vi "Time Left Calc.vi"(7 "Enum":T1, 8 "error in (no error)":errorcluster, 11 "Time":u32) -> (0 "error out":errorcluster, 2 "Time Left":u32, 3 "Total time":u32)   [LabVIEW 2018]
uses:
  Time elapsed.ctl
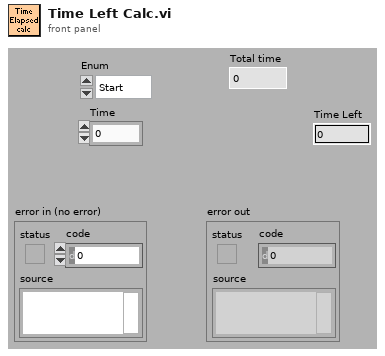
[diagram p1: front panel]
types:
  T1 = typedef "Time elapsed.ctl" = enum16{"Start", "Update", "Read"}
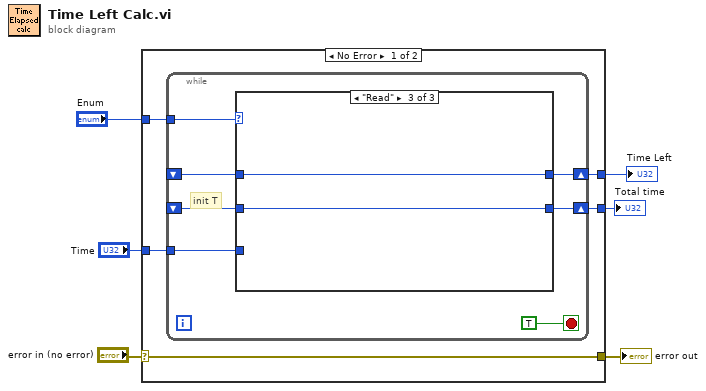
[diagram p0: block diagram]
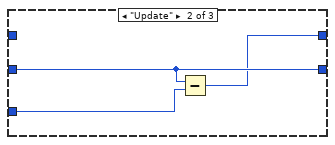
[diagram p3: hidden frame]
diagram:
  n1 = case shown="No Error" "error in (no error)" {
    selector: "error in (no error)" -> [w11 w25]
    tunnel: [w11 w25] -> w5
    tunnel: "Time" -> [w10 _]
    tunnel: [w9 _] -> w3
    tunnel: "Enum" -> [w8 _]
    tunnel: [w7 _] -> w1
    frame No Error {
      n2 = while {
        shift-right: [w12] -> w7
        shift-left: _ -> [w17]
        tunnel: w10 -> [w16]
        tunnel: w8 -> [w14]
        shift-right: [w15] -> w9
        shift-left: _ -> [w13]
        stop <- TRUE stop-if-true
        # "init T"
        n3 = case shown="\"Read\"" w14 {
          tunnel: [w19 w22 w23] -> w12
          tunnel: w17 -> [_ w22 w23]
          tunnel: w16 -> [w19 w21 _]
          tunnel: [w19 w20 w24] -> w15
          tunnel: w13 -> [_ _ w24]
          frame "Start" {
          }
          frame "Update" {
            n4 = Subtract(x=w22, y=w21) -> (x-y=w20:u32)
          }
          frame "Read" {
          }
        }
      }
    }
    frame Error {
    }
  }
  "error out" <- w5
  "Time Left" <- w3
  "Total time" <- w1
